vi "Write Bandwidth (nm).vi"(8 "error in (no error)":errorcluster, 10 "Bandwidth (nm)":dbl, 11 "Light Source in":refnum<class "Light Source.lvclass">) -> (0 "error out":errorcluster, 3 "Light Source out":refnum<class "Light Source.lvclass">)   [LabVIEW 2017, in "Light Source.lvclass"]
uses:
  Light Source.lvclass
  Light Source.lvclass/Light Source.ctl
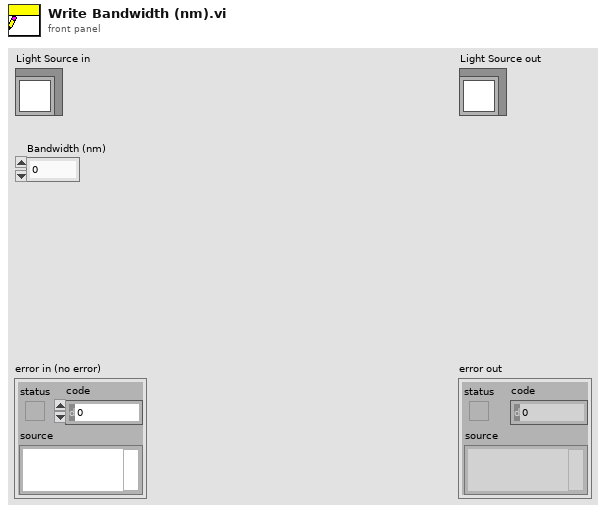
[diagram p1: front panel]
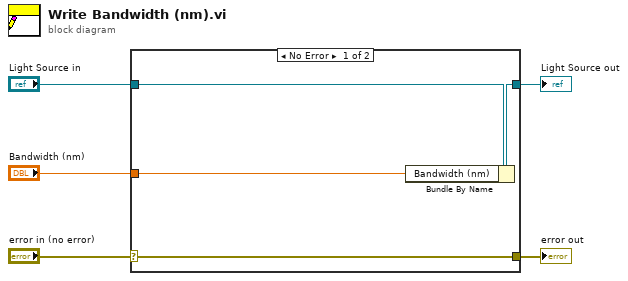
[diagram p0: block diagram]
diagram:
  n1 = case shown="No Error" "error in (no error)" {
    selector: "error in (no error)" -> [w9 w10]
    tunnel: [w9 w10] -> w4
    tunnel: [w7 w11] -> w2
    tunnel: "Light Source in" -> [w8 w11]
    tunnel: "Bandwidth (nm)" -> [w6 _]
    frame No Error {
      n2 = Bundle By Name(cluster=w8, "Bandwidth (nm)"=w6) -> (w7:refnum<class "Light Source.lvclass">)
    }
    frame Error {
    }
  }
  "error out" <- w4
  "Light Source out" <- w2
